vi "CRYAppend rep # prefixes.vi"(11 "Curves list in":string[](array[string])) -> (3 "Curves list with no repeats":string[](array[string]))   [LabVIEW 2013]
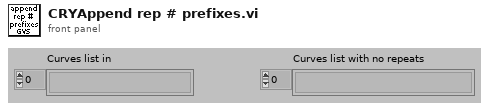
[diagram p1: front panel]
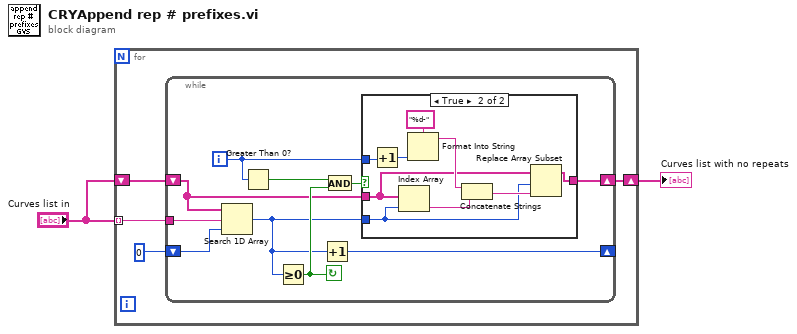
[diagram p0: block diagram]
diagram:
  n1 = for {
    tunnel: "Curves list in" -> [w6] mode=indexing
    shift-right: [w4] -> w1
    shift-left: "Curves list in" -> [w3]
    n2 = while {
      shift-left: w3 -> [w7]
      shift-right: [w8] -> w4
      shift-left: 0 -> [w15]
      shift-right: [w14] -> _
      tunnel: w6 -> [w16]
      i -> [w10]
      stop <- w12 continue-if-true
      n3 = Search 1D Array(1D array=w7, element=w16, start index (0)=w15) -> (index of element=w9:i32)
      n4 = Greater Than 0?(x=w10) -> (x > 0?=w13:bool)
      n5 = Greater Or Equal To 0?(x=w9) -> (x >= 0?=w12:bool)
      n6 = Increment(x=w9) -> (x+1=w14:i32)
      n7 = And(x=w13, y=w12) -> (x .and. y?=w11:bool)
      n8 = case shown="True" w11 {
        tunnel: w7 -> [w17 w19]
        tunnel: w10 -> [_ w26]
        tunnel: w9 -> [_ w20]
        tunnel: [w17 w18] -> w8
        frame False {
        }
        frame True {
          n9 = Increment(x=w26) -> (x+1=w25:i32)
          n10 = Index Array(array=w19, index=w20) -> (element=w23:string)
          n11 = Format Into String(format string="%d-", w25) -> (resulting string=w22:string)  [unwired: 2 in, 1 out]
          n12 = Concatenate Strings(w22, w23) -> (w21:string)
          n13 = Replace Array Subset(array=w19, new element=w21, index=w20) -> (w18:string[])
        }
      }
    }
  }
  "Curves list with no repeats" <- w1
